vi "Kommunikation Loopkennung.vi"(8 "error in (no error)":errorcluster caption="Fehler (Eingang, kein Fehler)", 10 "PNS SprachIndex (Seite)":i32=24, 11 "Steuerung PNS Eingang":refnum<class "Steuerung PNS.lvclass">) -> (0 "error out":errorcluster caption="Fehler (Ausgang)", 1 "Loopkennung":u16[](array[numeric]), 2 "Loops":string[](array[string]), 3 "Steuerung PNS Ausgang":refnum<class "Steuerung PNS.lvclass">)   [LabVIEW 2020, in "Steuerung PNS.lvclass"]
doc: "Kommuniziert mit der Steuerung, um die LoopKennungen auszulesen und in mehrsprachigen Text umzuwandeln, speichert diese im Objekt und stellt sie gleichzeitig als Output zur Verfügung.\nRIW"
uses:
  Steuerung PNS.lvclass
  Steuerung PNS.lvclass/Steuerung PNS.ctl
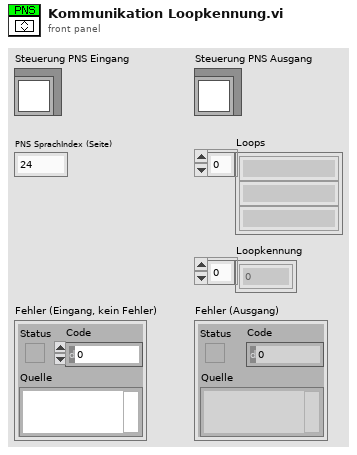
[diagram p1: front panel]
types:
  T1 = typedef "Steuerung PNS.lvclass/Adresse.ctl" = cluster{i32[][], i32}
  T2 = typedef "Steuerung PNS.lvclass/Werte.ctl" = cluster{"Adressen":u16[], "Werte":u16[]}
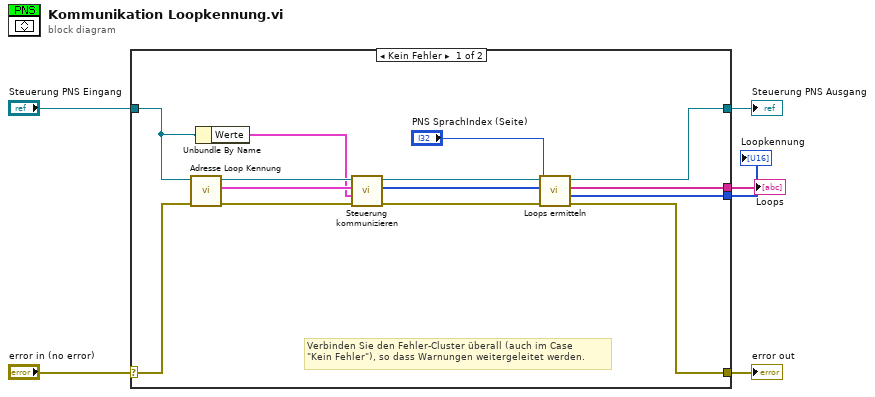
[diagram p0: block diagram]
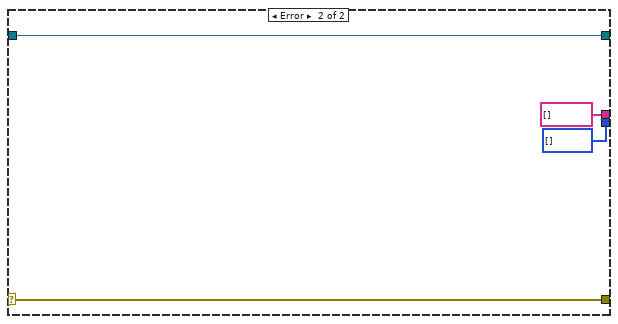
[diagram p2: hidden frame]
diagram:
  n1 = case shown="Kein Fehler" "error in (no error)" {
    selector: "error in (no error)" -> [w14 w24]
    tunnel: [w13 w24] -> w5
    tunnel: [w11 w23] -> w3
    tunnel: "Steuerung PNS Eingang" -> [w12 w23]
    tunnel: [w10 string[] [] ("Loops")] -> w2
    tunnel: [w8 u16[] [] ("Loopkennung")] -> w1
    frame No Error {
      # "Verbinden Sie den Fehler-Cluster überall (auch im Case\n\"Kein Fehler\"), so dass Warnungen weitergeleitet werden."
      n2 = call-dynamic "Adresse Loop Kennung.vi"("error in (no error)"=w14, "Steuerung PNS Eingang"=w12) -> ("error out"=w19:errorcluster, "Adressen"=w18:T1, "Steuerung PNS Ausgang"=w20:refnum<class "Steuerung PNS.lvclass">)  [unwired: 7 in]
      n3 = Unbundle By Name(w12) -> ("Werte"=w17:T2)
      n4 = call "Steuerung kommunizieren.vi"("Steuerung PNS Eingang"=w20, "Adressen"=w18, "Werte"=w17, "error in (no error)"=w19) -> ("Steuerung PNS Ausgang"=w16:refnum<class "Steuerung PNS.lvclass">, "Istwerte"=w9:u16[], "error out"=w15:errorcluster)  [unwired: 4 in]
      n5 = call "Loops ermitteln.vi"("error in (no error)"=w15, "PNS SprachIndex (Seite)"="PNS SprachIndex (Seite)", "Istwerte"=w9, "Steuerung PNS Eingang"=w16) -> ("error out"=w13:errorcluster, "Loopkennung"=w8:u16[], "Loops"=w10:string[], "Steuerung PNS Ausgang"=w11:refnum<class "Steuerung PNS.lvclass">)  [unwired: 4 in]
    }
    frame Error {
    }
  }
  "error out" <- w5
  "Steuerung PNS Ausgang" <- w3
  "Loops" <- w2
  "Loopkennung" <- w1
